vi "PPSU FGV.vi"(8 "error in":errorcluster, 9 "PPSU (W)":T1, 11 "Write/Read":T2=enum."Read") -> (0 "error out":errorcluster, 1 "PPSU (R)":T1)   [LabVIEW 2022 SP3]
uses:
  Controls/FGV Read write.ctl
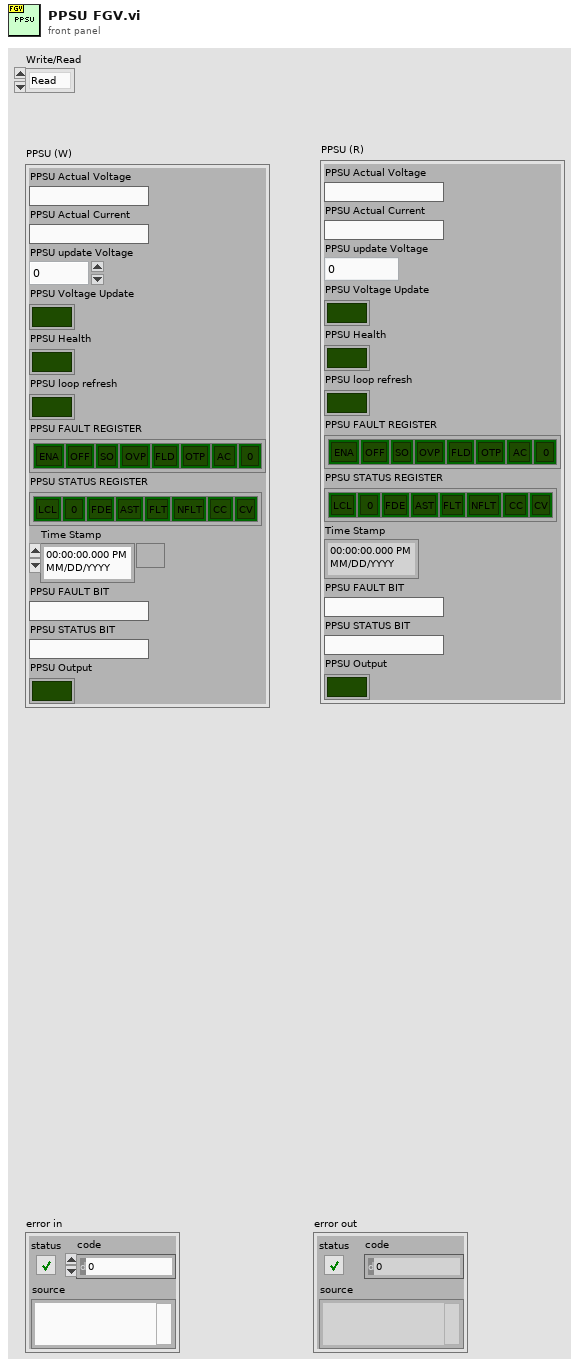
[diagram p1: front panel]
types:
  T1 = cluster{"PPSU Actual Voltage ":string, "PPSU Actual Current ":string, "PPSU update Voltage ":dbl, "PPSU Voltage Update":bool, "PPSU Health":bool, "PPSU loop refresh":bool, "PPSU FAULT REGISTER":cluster{"[0]":bool, "[1]":bool, "[2]":bool, "[3]":bool, "[4]":bool, "[5]":bool, "[6]":bool, "[7]":bool, "[8]":bool}, "PPSU STATUS REGISTER":cluster{"[0]":bool, "[1]":bool, "[2]":bool, "[3]":bool, "[4]":bool, "[5]":bool, "[6]":bool, "[7]":bool, "[8]":bool}, "Time Stamp":timestamp, "PPSU FAULT BIT":string, "PPSU STATUS BIT ":string, "PPSU Output":bool}
  T2 = typedef "FGV Read write.ctl" = enum16{"Write", "Read"}
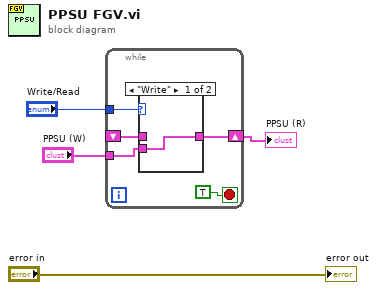
[diagram p0: block diagram]
diagram:
  n1 = while {
    tunnel: "Write/Read" -> [w8]
    shift-right: [w7] -> w1
    shift-left: _ -> [w6]
    tunnel: "PPSU (W)" -> [w5]
    stop <- TRUE stop-if-true
    n2 = case shown="\"Write\"" w8 {
      tunnel: [w10 w11] -> w7
      tunnel: w6 -> [_ w11]
      tunnel: w5 -> [w10 _]
      frame "Write" {
      }
      frame "Read" {
      }
    }
  }
  "PPSU (R)" <- w1
  "error out" <- "error in"
